vi "Get Static Methods in LVClass.vi"(8 "error in (no error)":errorcluster, 11 "LVClassLibrary in":refnum<vi>) -> (0 "error out":errorcluster, 2 "Static Member VIs[]":refnum<vi>[](array[refnum]), 3 "LVClassLibrary out":refnum<vi>)   [LabVIEW 2019, in "gRPC Template Creation Utility.lvlib"]
uses:
  gRPC Template Creation Utility.lvlib
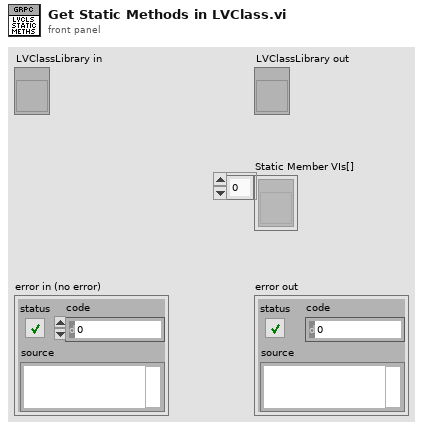
[diagram p1: front panel]
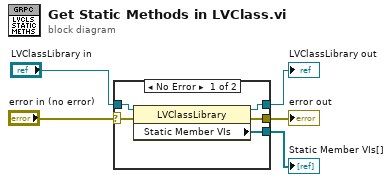
[diagram p0: block diagram]
diagram:
  n1 = case shown="No Error" "error in (no error)" {
    selector: "error in (no error)" -> [w6 w12]
    tunnel: "LVClassLibrary in" -> [w10 w11]
    tunnel: [w9 w11] -> w4
    tunnel: [w8 w12] -> w3
    tunnel: [w7 _] -> w2
    frame No Error {
      n2 = property class="LVClassLibrary"(reference=w10, error in=w6) -> (reference out=w9:refnum<vi>, error out=w8:errorcluster, "Static Member VIs"=w7:refnum<vi>[])
    }
    frame Error {
    }
  }
  "LVClassLibrary out" <- w4
  "error out" <- w3
  "Static Member VIs[]" <- w2
